vi "DAQ_TTC Meas Initialize.vi"(0 "Physical Channels":tag, 5 "Global Channels":refnum<k21>, 7 "CJC Source":i32(ring)=10200 items=["Built-In"=10200, "Constant Value"=10116, "Channel"=10113], 9 "CJC Channel":refnum<k21>, 11 "error in":errorcluster) -> (4 "DAQmx Task Out":refnum<k21>, 15 "error out":errorcluster)   [LabVIEW 2021, in "DAQ_Temperature Thermocouple Measurement.lvlib"]
doc: "Initialize analog input channels for Temperature Thermocouple and obtains a DAQmx task\n\nProvide either Physical channel or Global Channel.\nIf both physical and Global channels are provided, Global Channels will take precedence\n\nNote: For Physical Channel selection, CJC Source and CJC Channel must be configured."
uses:
  DAQ_Temperature Thermocouple Measurement.lvlib
  <vilib>/DAQmx/create/channels.llb/DAQmx Create Channel (AI-Temperature-Thermocouple).vi
panel:
  # "Inputs"
  # "Outputs"
  # "Overview:\nThis VI initializes NI cDAQ AI Module and provides the DAQmx Task Out\n\nHardware Requirements: NI C Series/cDAQ Temperature Input Module (Ex: NI-9211)\n\nSoftware Requirements: NI DAQmx 2022 Q4 or later\n\nInstructions:\n1. Enter physical channel in which Temparature Measurement has to be done in Physical Channels control (Or) Enter Global channels to use it instead of initiating a new task. User must configure only one input. If both are provided, Global Channels will take precedence.\n2. Specify CJC Source type and CJC Channel to use for Cold junction compensation. Uses a global channel or another virtual channel already in the task.\n3. Get the Temperature Thermocouple Measurement task from DAQmx Task Out.\n\nNote: User can use the DAQmx Task on other modules to configure and initiate Temparature Thermocouple Measurements."
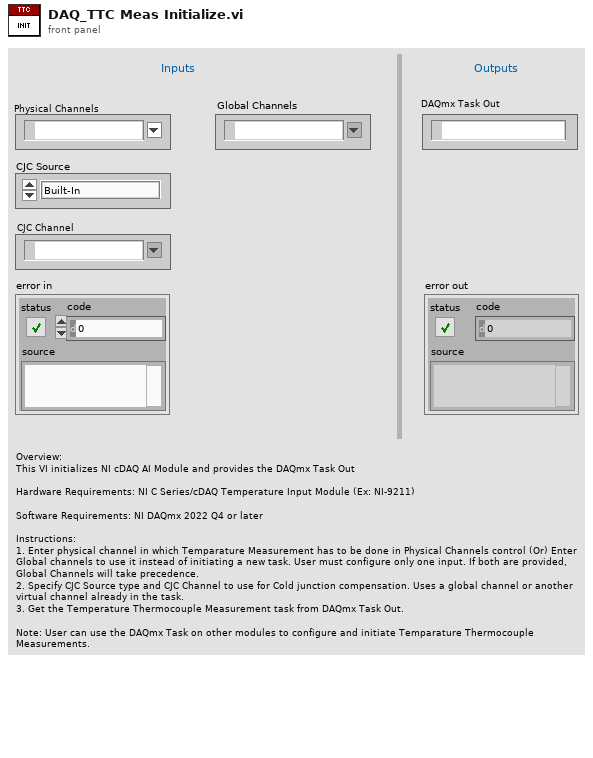
[diagram p1: front panel]
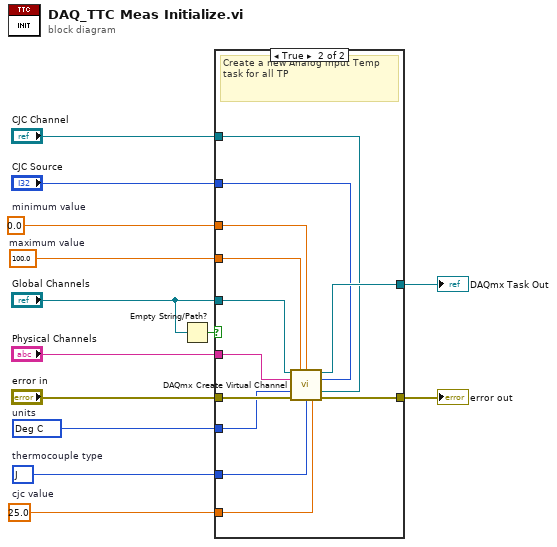
[diagram p0: block diagram]
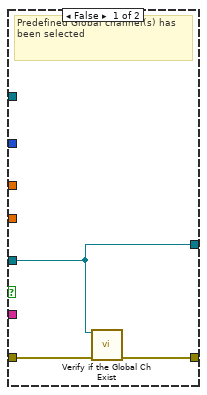
[diagram p2: hidden frame]
diagram:
  w4 = 100.0  # maximum value
  w3 = 0.0  # minimum value
  w6 = 25.0  # cjc value
  w5 = 10072 items=["J"=10072, "K"=10073, "N"=10077, "R"=10082, "S"=10085, "T"=10086, "B"=10047, "E"=10055]  # thermocouple type
  w7 = 10143 items=["Deg C"=10143, "Deg F"=10144, "Kelvins"=10325, "Deg R"=10145, "From Custom Scale"=10065]  # units
  n1 = Empty String/Path?(string/path="Global Channels") -> (empty?=w9:bool)
  n2 = case shown="True" w9 {
    tunnel: "Physical Channels" -> [_ w26]
    tunnel: "Global Channels" -> [w14 w17]
    tunnel: [w14 w28] -> w10
    tunnel: "error in" -> [w16 w27]
    tunnel: [w15 w25] -> w13
    tunnel: w7 -> [_ w24]
    tunnel: "CJC Source" -> [_ w23]
    tunnel: "CJC Channel" -> [_ w22]
    tunnel: w6 -> [_ w21]
    tunnel: w5 -> [_ w20]
    tunnel: w4 -> [_ w19]
    tunnel: w3 -> [_ w18]
    frame False {
      # "Predefined Global channel(s) has been selected"
      n3 = call "Verify if the Global Ch Exist.vi"("Global Channels"=w14, "error in (no error)"=w16) -> ("error out"=w15:errorcluster)  [unwired: 13 in]
    }
    frame True {
      # "Create a new Analog input Temp task for all TP"
      n4 = call-poly <vilib>:"DAQmx Create Virtual Channel.vi"("task in"=w17, "maximum value"=w19, "minimum value"=w18, "physical channels"=w26, "cjc source"=w23, "units"=w24, "cjc channel"=w22, "error in"=w27, "thermocouple type"=w20, "cjc value"=w21) -> ("task out"=w28:refnum<k21>, "error out"=w25:errorcluster)  [unwired: 4 in]
    }
  }
  "DAQmx Task Out" <- w10
  "error out" <- w13
